vi "两板卡同步_参考时钟同步_主卡内部触发.vi"() -> ()   [LabVIEW 2013]
doc: "This example demonstrates how to acquire a continuous data."
uses:
  <userlib>/ArtDAQ/_SubVI/ArtDAQ_CreateAIVoltageIEPEChan.vi
  <userlib>/ArtDAQ/_SubVI/ArtDAQ_CfgSampClkTiming.vi
  <userlib>/ArtDAQ/_SubVI/ArtDAQ_CfgDigEdgeStartTrig.vi
  <userlib>/ArtDAQ/_SubVI/ArtDAQ_Read Analog DBL NChan NSamp.vi
panel:
  in  "从卡触发接入端":string="RTSI9"
  in  "主卡触发导出端":string="RTSI9"
  in  "从卡参考时钟源":string="RTSI9"
  in  "主卡参考时钟源":string="RTSI9"
  in  "从卡物理通道":string(combo)="Dev1/ai0"
  out "从卡波形图":dbl[][](graph)
  in  "停止":bool
  out "主卡波形图":dbl[][](graph)
  in  "采样速率":dbl=10000.0 format="%#_13g"
  in  "主卡物理通道":string(combo)="Dev1/ai0"
  out "错误":errorcluster
  # "通道属性"
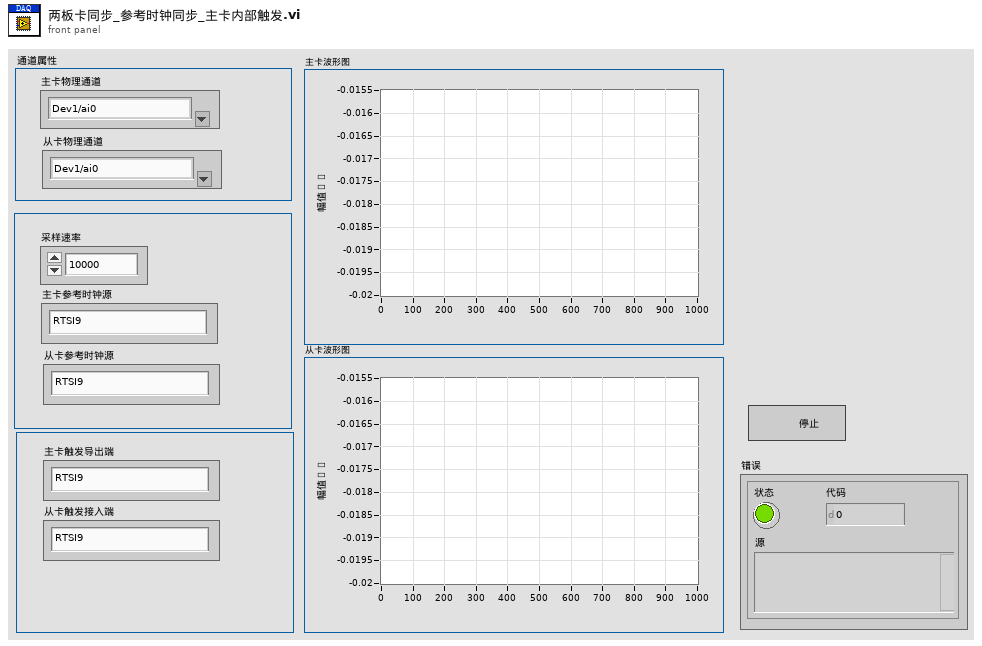
[diagram p1: front panel]
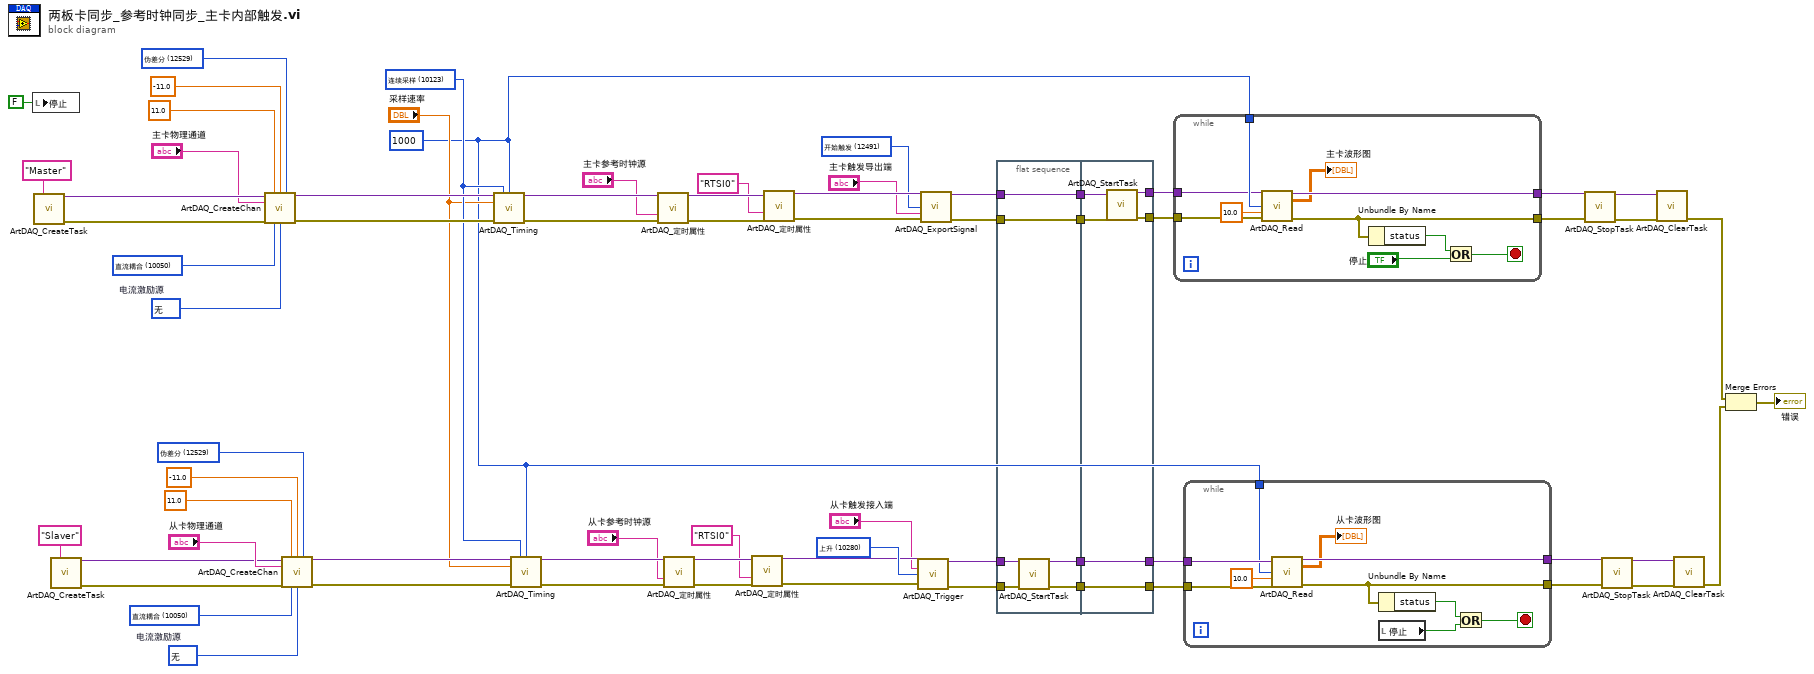
[diagram p0: block diagram]
diagram:
  w32 = 10280 items=["上升"=10280, "下降"=10171] ("斜率 2")
  w13 = 12491 items=["AI转换时钟"=12484, "10MHz参考时钟"=12536, "20MHz时基时钟"=12486, "采样时钟"=12487, "前移触发"=12488, "参考触发"=12490, "开始触发"=12491] ("信号")
  w33 = 1000 ("每通道采样数 2")
  w52 = 10050 items=["交流耦合"=10045, "直流耦合"=10050, "接地"=10066] ("耦合 2")
  w57 = 10050 items=["交流耦合"=10045, "直流耦合"=10050, "接地"=10066] ("耦合")
  w39 = 12529 items=["默认"=-1, "单端"=10083, "非参考单端"=10078, "差分"=10106, "伪差分"=12529] ("接线端配置 2")
  w66 = 12529 items=["默认"=-1, "单端"=10083, "非参考单端"=10078, "差分"=10106, "伪差分"=12529] ("接线端配置")
  w53 = 10230 items=["内部"=10200, "外部"=10167, "无"=10230]  # 电流激励源
  w35 = 10123 items=["有限点采样"=10178, "连续采样"=10123] ("SampleMode")
  w56 = 10230 items=["内部"=10200, "外部"=10167, "无"=10230]  # 电流激励源
  n1 = local write "停止"(FALSE ("停止")) -> ()
  n2 = call <userlib>:"ArtDAQ_CreateTask.vi"("任务名称"="Master") -> ("任务句柄"=w64:variant, "错误输出"=w69:errorcluster)  [unwired: 13 in]
  n3 = call <userlib>:"ArtDAQ_CreateTask.vi"("任务名称"="Slaver") -> ("任务句柄"=w43:variant, "错误输出"=w36:errorcluster)  [unwired: 13 in]
  n4 = call-poly <userlib>:"ArtDAQ_CreateChan.vi"("任务句柄"=w64, "最大值"=11.0 ("最大值(V)"), "最小值"=-11.0 ("最小值(V)"), "接线端配置"=w66, "物理通道"="主卡物理通道", "错误输入"=w69, "耦合方式"=w57, "电流激励源"=w56) -> ("任务句柄"=w58:variant, "错误输出"=w65:errorcluster)  [unwired: 6 in]
  n5 = call-poly <userlib>:"ArtDAQ_CreateChan.vi"("任务句柄"=w43, "最大值"=11.0 ("最大值(V) 2"), "最小值"=-11.0 ("最小值(V) 2"), "接线端配置"=w39, "物理通道"="从卡物理通道", "错误输入"=w36, "耦合方式"=w52, "电流激励源"=w53) -> ("任务句柄"=w51:variant, "错误输出"=w40:errorcluster)  [unwired: 6 in]
  n6 = call-poly <userlib>:"ArtDAQ_Timing.vi"("任务句柄"=w58, "采样模式"=w35, "每通道采样数"=w33, "采样率"="采样速率", "错误输入"=w65) -> ("任务句柄"=w28:variant, "错误输出"=w27:errorcluster)  [unwired: 9 in]
  n7 = call-poly <userlib>:"ArtDAQ_Timing.vi"("任务句柄"=w51, "采样模式"=w35, "每通道采样数"=w33, "采样率"="采样速率", "错误输入"=w40) -> ("任务句柄"=w26:variant, "错误输出"=w25:errorcluster)  [unwired: 9 in]
  n8 = call-poly "ArtDAQ_定时属性.vi"("任务句柄"=w28, "参考时钟源"="主卡参考时钟源", "错误输入"=w27) -> ("任务句柄"=w22:variant, "错误输出"=w23:errorcluster)  [unwired: 11 in]
  n9 = call-poly "ArtDAQ_定时属性.vi"("任务句柄"=w26, "参考时钟源"="从卡参考时钟源", "错误输入"=w25) -> ("任务句柄"=w20:variant, "错误输出"=w19:errorcluster)  [unwired: 11 in]
  n10 = call-poly "ArtDAQ_定时属性.vi"("任务句柄"=w20, "同步脉冲源"="RTSI0", "错误输入"=w19) -> ("任务句柄"=w17:variant, "错误输出"=w18:errorcluster)  [unwired: 11 in]
  n11 = call-poly "ArtDAQ_定时属性.vi"("任务句柄"=w22, "同步脉冲源"="RTSI0", "错误输入"=w23) -> ("任务句柄"=w15:variant, "错误输出"=w14:errorcluster)  [unwired: 11 in]
  n12 = call-poly <userlib>:"ArtDAQ_Trigger.vi"("任务句柄"=w17, "触发源"="从卡触发接入端", "边沿"=w32, "错误输入"=w18) -> ("任务句柄"=w48:variant, "错误输出"=w49:errorcluster)  [unwired: 10 in]
  n13 = call <userlib>:"ArtDAQ_ExportSignal.vi"("任务句柄"=w15, "信号"=w13, "输出接线端"="主卡触发导出端", "错误输入"=w14) -> ("任务句柄"=w10:variant, "错误输出"=w8:errorcluster)  [unwired: 10 in]
  n14 = flat-sequence {
    tunnel: w49 -> [w75]
    tunnel: w48 -> [w74]
    tunnel: [w73] -> w12
    tunnel: [w72] -> w11
    tunnel: w10 -> [w71]
    tunnel: [w71] -> w9
    tunnel: w8 -> [w70]
    tunnel: [w70] -> w7
    tunnel: [w80] -> w41
    tunnel: [w81] -> w42
    tunnel: w12 -> [w81]
    tunnel: w11 -> [w80]
    tunnel: w9 -> [w79]
    tunnel: w7 -> [w78]
    tunnel: [w77] -> w6
    tunnel: [w76] -> w5
    frame #0 {
      n15 = call <userlib>:"ArtDAQ_StartTask.vi"("任务句柄"=w74, "错误输入"=w75) -> ("任务句柄"=w72:variant, "错误输出"=w73:errorcluster)  [unwired: 12 in]
    }
    frame #1 {
      n16 = call <userlib>:"ArtDAQ_StartTask.vi"("任务句柄"=w79, "错误输入"=w78) -> ("任务句柄"=w77:variant, "错误输出"=w76:errorcluster)  [unwired: 12 in]
    }
  }
  n17 = while {
    tunnel: w33 -> [w91]
    tunnel: [w89] -> w63
    tunnel: [w88] -> w62
    tunnel: w6 -> [w83]
    tunnel: w5 -> [w82]
    stop <- w86 stop-if-true
    n18 = call-poly <userlib>:"ArtDAQ_Read.vi"("任务句柄"=w83, "每通道采样数"=w91, "超时s"=10.0 ("Timeout"), "错误输入"=w82) -> ("任务句柄"=w89:variant, "数据"=→"主卡波形图":dbl[][], "错误输出"=w88:errorcluster)  [unwired: 8 in, 1 out]
    n19 = Unbundle By Name(w88) -> ("status"=w87:bool)
    n20 = Or(x=w87, y="停止") -> (x .or. y?=w86:bool)
  }
  n21 = while {
    tunnel: w41 -> [w101]
    tunnel: w42 -> [w100]
    tunnel: w33 -> [w99]
    tunnel: [w97] -> w44
    tunnel: [w96] -> w45
    stop <- w93 stop-if-true
    n22 = call-poly <userlib>:"ArtDAQ_Read.vi"("任务句柄"=w101, "每通道采样数"=w99, "超时s"=10.0 ("Timeout"), "错误输入"=w100) -> ("任务句柄"=w97:variant, "数据"=→"从卡波形图":dbl[][], "错误输出"=w96:errorcluster)  [unwired: 8 in, 1 out]
    n23 = Unbundle By Name(w96) -> ("status"=w95:bool)
    n24 = local read "停止"() -> (w92:bool)
    n25 = Or(x=w95, y=w92) -> (x .or. y?=w93:bool)
  }
  n26 = call <userlib>:"ArtDAQ_StopTask.vi"("任务句柄"=w63, "错误输入"=w62) -> ("任务句柄"=w61:variant, "错误输出"=w60:errorcluster)  [unwired: 12 in]
  n27 = call <userlib>:"ArtDAQ_StopTask.vi"("任务句柄"=w44, "错误输入"=w45) -> ("任务句柄"=w46:variant, "错误输出"=w47:errorcluster)  [unwired: 12 in]
  n28 = call <userlib>:"ArtDAQ_ClearTask.vi"("任务句柄"=w61, "错误输入"=w60) -> ("错误输出"=w31:errorcluster)  [unwired: 13 in]
  n29 = call <userlib>:"ArtDAQ_ClearTask.vi"("任务句柄"=w46, "错误输入"=w47) -> ("错误输出"=w30:errorcluster)  [unwired: 13 in]
  n30 = Merge Errors(w31, w30) -> (→"错误":errorcluster)
